vi "_Write Server Control.vi"(4 "Command":T2=enum."Start Run", 5 "Text":string, 6 "error in (no error)":errorcluster, 7 "Boolean (F)":bool, 8 "Control Type":T1, 9 "Control Ref":refnum<vi>) -> (0 "error out":errorcluster)   [LabVIEW 2015]
uses:
  Type/_Server Command.ctl
  Type/_Server Control Type.ctl
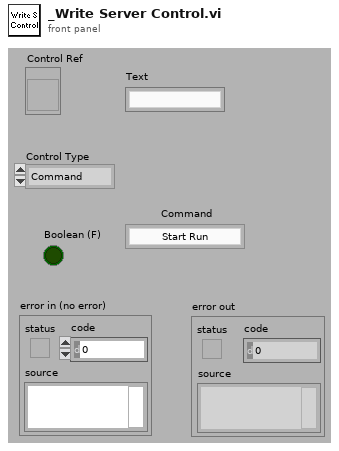
[diagram p1: front panel]
types:
  T1 = typedef "_Server Control Type.ctl" = enum16{"Command", "Boolean", "Text"}
  T2 = typedef "_Server Command.ctl" = enum16{"Hide Server", "Show Server", "Close Server", "Start Run", "Start Actual Run", "Stop Run", "Runtime Update", "Get Data", "Get Status", "Get Table", "Set Table", "Get Configuration", "Reserved", "Get Memory Map", "Read ADC", "Set Oscillator", "Reboot", "Backup Firmware", "Update Firmware", "Auxiliary Update", "System Status", "Start System", "Shutdown System", "Start LC Equilibration", "Get LC Status", "Get LC Configuration", "Get LC Method Contents", "Rinse Autosampler", "Pump OnOff", "Oven OnOff", "Get LC Error", "Clear LC Error", "Set LC Input Logic", "Set LC Hold Logic", "Lock Server", "Get Current Method", "Get Real Time Data", "Connect LC", "Disconnect LC"}
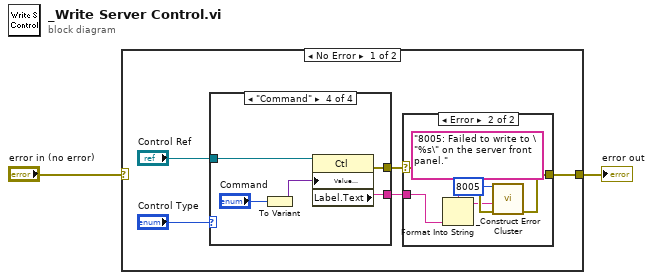
[diagram p0: block diagram]
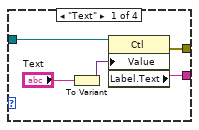
[diagram p2: hidden frame]
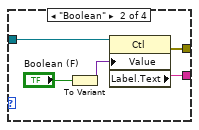
[diagram p3: hidden frame]
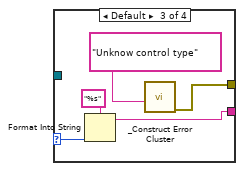
[diagram p4: hidden frame]
diagram:
  n1 = case shown="No Error" "error in (no error)" {
    selector: "error in (no error)" -> [_ w34]
    tunnel: [w7 w34] -> w1
    frame No Error {
      n2 = case shown="\"Command\"" "Control Type" {
        selector: "Control Type" -> [_ _ w20 _]
        tunnel: [w12 w14 w22 w25] -> w6
        tunnel: "Control Ref" -> [w11 w15 _ w26]
        tunnel: [w8 w13 w18 w23] -> w3
        frame "Text" {
          n3 = To Variant(anything="Text") -> (Variant=w9:variant)
          n4 = property class="Ctl"(reference=w11, "Value"=w9) -> (error out=w12:errorcluster, "Label.Text"=w8:string)  [unwired: 1 in, 1 out]
        }
        frame "Boolean" {
          n5 = To Variant(anything="Boolean (F)") -> (Variant=w16:variant)
          n6 = property class="Ctl"(reference=w15, "Value"=w16) -> (error out=w14:errorcluster, "Label.Text"=w13:string)  [unwired: 1 in, 1 out]
        }
        frame Default {
          n7 = Format Into String(format string="%s", w20) -> (resulting string=w18:string)  [unwired: 2 in, 1 out]
          n8 = call "_Construct Error Cluster.vi"("reason"="Unknow control type") -> ("error out"=w22:errorcluster)  [unwired: 3 in, 3 out]
        }
        frame "Command" {
          n9 = To Variant(anything="Command") -> (Variant=w27:variant)
          n10 = property class="Ctl"(reference=w26, "Value (Signaling)"=w27) -> (error out=w25:errorcluster, "Label.Text"=w23:string)  [unwired: 1 in, 1 out]
        }
      }
      n11 = case shown="Error" w6 {
        selector: w6 -> [_ w33]
        tunnel: [_ w30] -> w7
        tunnel: w3 -> [_ w29]
        frame No Error {
        }
        frame Error {
          n12 = Format Into String(format string="8005: Failed to write to \"%s\" on the server front panel.", w29) -> (resulting string=w31:string)  [unwired: 2 in, 1 out]
          n13 = call "_Construct Error Cluster.vi"("error in"=w33, "reason"=w31, "errorCode"=8005) -> ("error out"=w30:errorcluster)  [unwired: 1 in, 3 out]
        }
      }
    }
    frame Error {
    }
  }
  "error out" <- w1
